vi "Start.vi"(8 "error in (no error)":errorcluster, 11 "Analog Output in":refnum<class "Analog output.lvclass">) -> (0 "error out":errorcluster, 3 "Analog Output out":refnum<class "Analog output.lvclass">)   [LabVIEW 2009, in "MicroDAQ.lvlib" / "Analog output.lvclass"]
doc: "Starts generation."
uses:
  <instrlib>/MicroDAQ/Channel/Analog Output/Analog output.lvclass
  <instrlib>/MicroDAQ/Channel/Analog Output/Analog output.lvclass/Analog output.ctl
  <instrlib>/MicroDAQ/Mlink library wraper/mlink.lvlib
  <instrlib>/MicroDAQ/Channel/Channel.lvclass
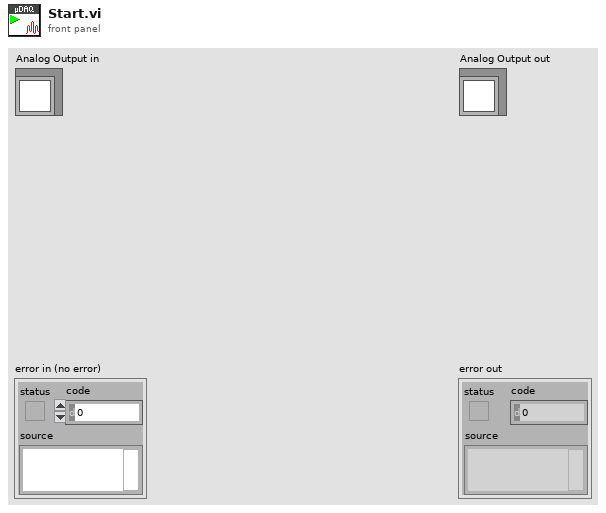
[diagram p1: front panel]
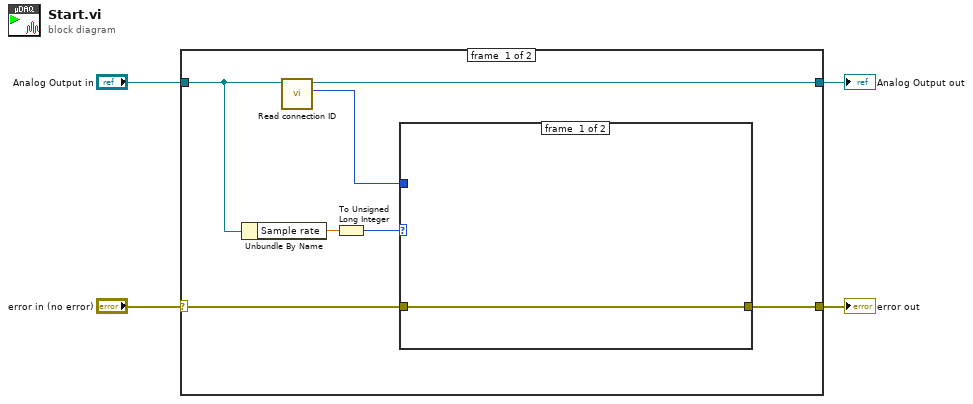
[diagram p0: block diagram]
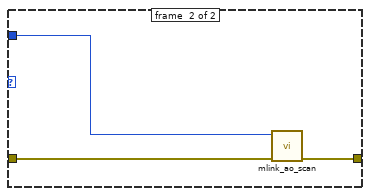
[diagram p2: hidden frame]
diagram:
  n1 = case shown="No Error" "error in (no error)" {
    selector: "error in (no error)" -> [w10 w16]
    tunnel: "Analog Output in" -> [w7 w17]
    tunnel: [w11 w16] -> w2
    tunnel: [w9 w17] -> w1
    frame #0 {
      n2 = Unbundle By Name(w7) -> ("Sample rate"=w6:dbl)
      n3 = call <instrlib>:"Read connection ID.vi"("Task in"=w7) -> ("connection ID"=w8:i32, "Task out"=w9:refnum<class "Analog output.lvclass">)  [unwired: 9 in]
      n4 = To Unsigned Long Integer(number=w6) -> (unsigned 32bit integer=w5:u32)
      n5 = case shown="Default" w5 {
        tunnel: [w12 w15] -> w11
        tunnel: w10 -> [w12 w14]
        tunnel: w8 -> [_ w13]
        frame #0 {
        }
        frame #1 {
          n6 = call <instrlib>:"mlink_ao_scan.vi"("error in (no error)"=w14, "connection ID"=w13) -> ("error out"=w15:errorcluster)  [unwired: 8 in, 1 out]
        }
      }
    }
    frame #1 {
    }
  }
  "error out" <- w2
  "Analog Output out" <- w1
